vi "Close_Instr.vi"(8 "error in (no error)":errorcluster caption="entrée d'erreur (pas d'erreur)", 11 "Class Instrument Patterm_Matching en entrée":refnum<class "Class Instrument Patterm_Matching.lvclass">) -> (0 "error out":errorcluster caption="sortie d'erreur", 3 "Class Instrument Patterm_Matching en sortie":refnum<class "Class Instrument Patterm_Matching.lvclass">)   [LabVIEW 2020, in "Library Instrument & Equipement.lvlib" / "Library Instruments.lvlib" / "Class Instrument Patterm_Matching.lvclass"]
doc: "releases and closes an instrument"
uses:
  Class Instrument Patterm_Matching.lvclass
  Class Instrument Patterm_Matching.lvclass/Class Instrument Patterm_Matching.ctl
  Camera/Class Camera Pattern Matching (Default)/Class Pattern Matching (Default).lvclass
  Instrument (Default)/Class Instrument (Default).lvclass
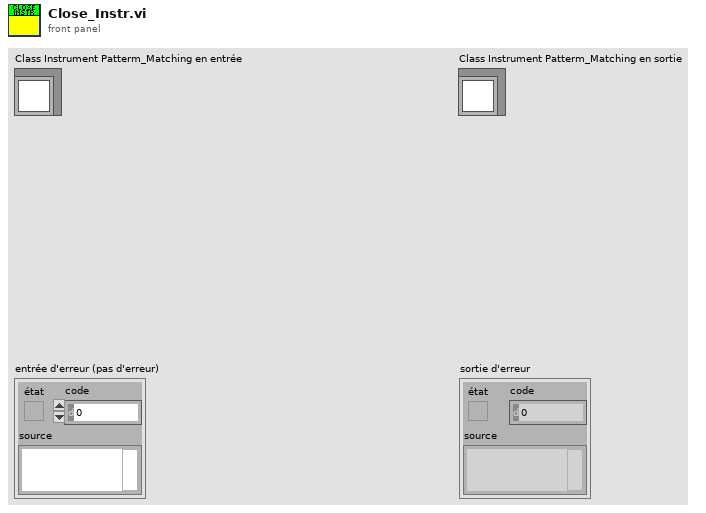
[diagram p1: front panel]
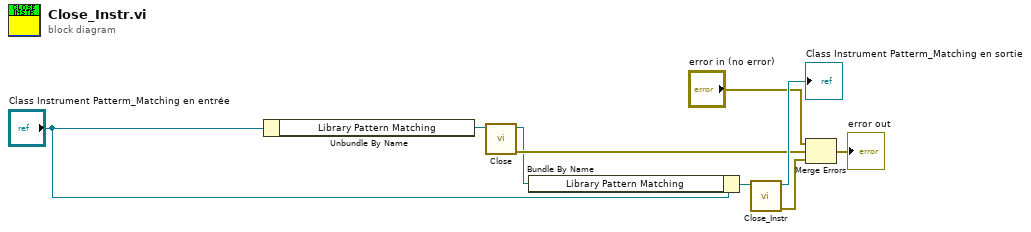
[diagram p0: block diagram]
diagram:
  n1 = Unbundle By Name("Class Instrument Patterm_Matching en entrée") -> ("Library Pattern Matching"=w4:refnum<class "Class Pattern Matching (Default).lvclass">)
  n2 = call-dynamic "Close.vi"("Class Camera IV3-500CA (Default) en entrée"=w4) -> ("error out"=w5:errorcluster, "Class Camera IV3-500CA (Default) en Sortie"=w1:refnum<class "Class Pattern Matching (Default).lvclass">)  [unwired: 9 in]
  n3 = Bundle By Name(cluster="Class Instrument Patterm_Matching en entrée", "Library Pattern Matching"=w1) -> (w2:refnum<class "Class Instrument Patterm_Matching.lvclass">)
  n4 = call-parent "Close_Instr.vi"("Class Instrument (Default) en entrée"=w2) -> ("error out"=w7:errorcluster, "Class Instrument (Default) en sortie"=→"Class Instrument Patterm_Matching en sortie":refnum<class "Class Instrument Patterm_Matching.lvclass">)  [unwired: 9 in]
  n5 = Merge Errors("error in (no error)", w5, w7) -> (→"error out":errorcluster)
